vi "ConvertVoltageToTemperature.vi"(1 "Voltage":dbl) -> (0 "Numérique":dbl)   [LabVIEW 2021]
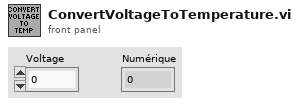
[diagram p1: front panel]
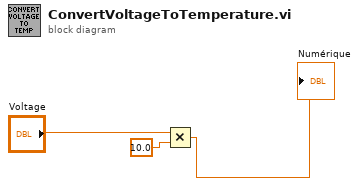
[diagram p0: block diagram]
diagram:
  n1 = Multiply(x="Voltage", y=10.0) -> (x*y=→"Numérique":dbl)
